vi "niFPGA BFGroup Twiddle Table 256 U64 Inv.vi"(7 "address":fxp<+,8,8>) -> (4 "twid real":fxp<+/-,33,2> format="%.32g", 6 "twid imag":fxp<+/-,33,2> format="%.32g")   [LabVIEW 2017]
uses:
  <vilib>/Utility/error.llb/Clear Errors.vi
  <vilib>/rvi/Emulation/niFpgaSctlEmulationGetInTimedLoop.vi
  <vilib>/rvi/DataTransferAndStorage/Container/Common/niFpgaContainerGetUniqueNameForEmu.vi
  <vilib>/rvi/DataTransferAndStorage/Container/Common/niFpgaContainerSetEmuInfo.vi
  <vilib>/rvi/eio/common/nirviEmuReportErrorAndStop.vi
  <vilib>/rvi/Memory/Memory_Emulation/nirvimemoryEmulation.vi
  <vilib>/rvi/Memory/Memory_Emulation/nirvimemoryFastEmulation.vi
  <vilib>/rvi/Memory/Memory_Emulation/niFpgaMemoryEmulationCacheClearOnFirstRun.vi
  <vilib>/rvi/Memory/Memory_Emulation/nirvimemoryEmulationManagerCache_MakeExclusive.vi
  <vilib>/rvi/Memory/Memory_Emulation/niFpgaMemoryEmulationValidateCache.vi
  <vilib>/rvi/Memory/Memory_Emulation/nirvimemoryEmulationManagerCache_InsertValue.vi
  <vilib>/rvi/Memory/Memory_Emulation/nirvimemoryEmulationManagerCache_ReleaseExclusive.vi
  <vilib>/rvi/Memory/Memory_Emulation/nirvimemoryEmulationManagerCache_GetValue.vi
  <vilib>/rvi/Emulation/niFpgaEmulationIsFPGAContextNoSignature.vi
  <vilib>/rvi/Memory/Memory_Emulation/nirvimemoryEmulationManagerCache_SetValue.vi
  <vilib>/rvi/Emulation/niFpgaSctlEmulationResourceMgr.vi
  <vilib>/rvi/LocalResourceManager/LocalResourceManager.xnode
  <vilib>/rvi/DataTransferAndStorage/Container/XNode/niFpgaContainer.xnode
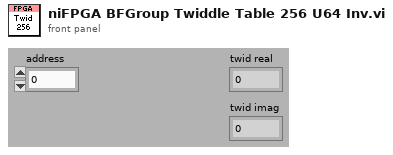
[diagram p1: front panel]
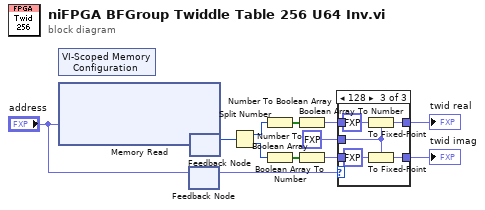
[diagram p0: block diagram]
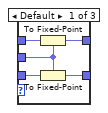
[diagram p2: hidden frame]
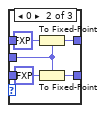
[diagram p3: hidden frame]
diagram:
  n1 = xnode "VI-Scoped Memory Configuration"() -> ()  [unwired: 1 out]
  n2 = xnode ("Memory Read")("Address"="address") -> ("Data"=w4:u64)  [unwired: 2 out]
  n3 = feedback-in #1("address") -> ()
  n4 = feedback #1() -> (w5:fxp<+,8,8>)  [unwired: 1 out]
  n5 = feedback-in #2(w4) -> ()
  n6 = feedback #2() -> (w9:u64)  [unwired: 1 out]
  n7 = Split Number(x=w9) -> (hi(x)=w12:u32, lo(x)=w10:u32)
  n8 = Number To Boolean Array(number=w12) -> (Boolean array=w13:bool[])
  n9 = Number To Boolean Array(number=w10) -> (Boolean array=w11:bool[])
  n10 = Boolean Array To Number(Boolean array=w13) -> (number=w7:fxp<+/-,32,1>)
  n11 = Boolean Array To Number(Boolean array=w11) -> (number=w6:fxp<+/-,32,1>)
  n12 = case shown="128" w5 {
    tunnel: w7 -> [w18 _ _]
    tunnel: [w17 w22 w27] -> w3
    tunnel: w6 -> [w16 _ _]
    tunnel: [w15 w21 w26] -> w2
    tunnel: fxp<+/-,33,2> 0.0 ("fixed-point type") -> [w14 w19 w24]
    frame Default {
      n13 = To Fixed-Point(fixed-point type=w14, number=w18) -> (fixed-point=w17:fxp<+/-,33,2>)
      n14 = To Fixed-Point(fixed-point type=w14, number=w16) -> (fixed-point=w15:fxp<+/-,33,2>)
    }
    frame 0 {
      n15 = To Fixed-Point(fixed-point type=w19, number=fxp<+,1,1> 1.0 ("fixed-point type")) -> (fixed-point=w22:fxp<+/-,33,2>)
      n16 = To Fixed-Point(fixed-point type=w19, number=fxp<+,1,1> 0.0 ("fixed-point type")) -> (fixed-point=w21:fxp<+/-,33,2>)
    }
    frame 128 {
      n17 = To Fixed-Point(fixed-point type=w24, number=fxp<+,1,1> 0.0 ("fixed-point type")) -> (fixed-point=w27:fxp<+/-,33,2>)
      n18 = To Fixed-Point(fixed-point type=w24, number=fxp<+,1,1> 1.0 ("fixed-point type")) -> (fixed-point=w26:fxp<+/-,33,2>)
    }
  }
  "twid real" <- w3
  "twid imag" <- w2
